vi "Initialize State.vi"(8 "error in (no error)":errorcluster, 11 "Elevator Controller in":refnum<class "Elevator Controller.lvclass">) -> (0 "error out":errorcluster, 3 "Elevator Controller out":refnum<class "Elevator Controller.lvclass">)   [LabVIEW 2019]
uses:
  Abstract Display Console Actor/Abstract Display Console Messages/Initialize Display State Msg/Initialize Display State Msg.lvclass
  Abstract Sensor Interface Actor/Abstract Sensor Interface Messages/Initalize Sensor Interface State Msg/Initalize Sensor Interface State Msg.lvclass
  Abstract User Console Actor/Abstract User Console Messages/Initialize User Console State Msg/Initialize User Console State Msg.lvclass
  <vilib>/ActorFramework/Message Enqueuer/Message Enqueuer.lvclass
  Elevator Controller.lvclass
  C:/Program Files (x86)/National Instruments/LabVIEW 2019/vi.lib/ActorFramework/Actor/Actor.lvclass
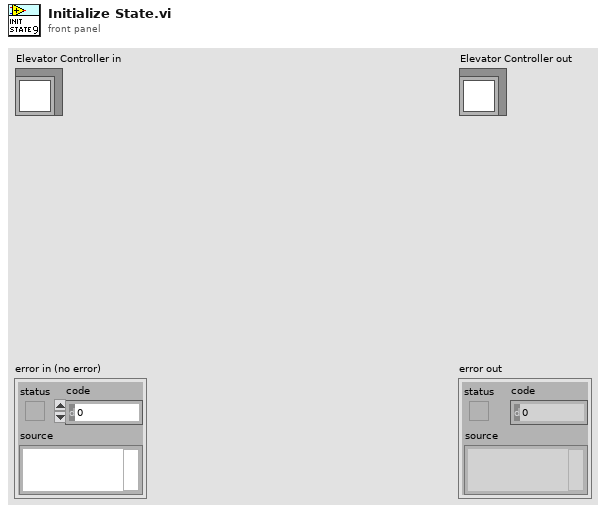
[diagram p1: front panel]
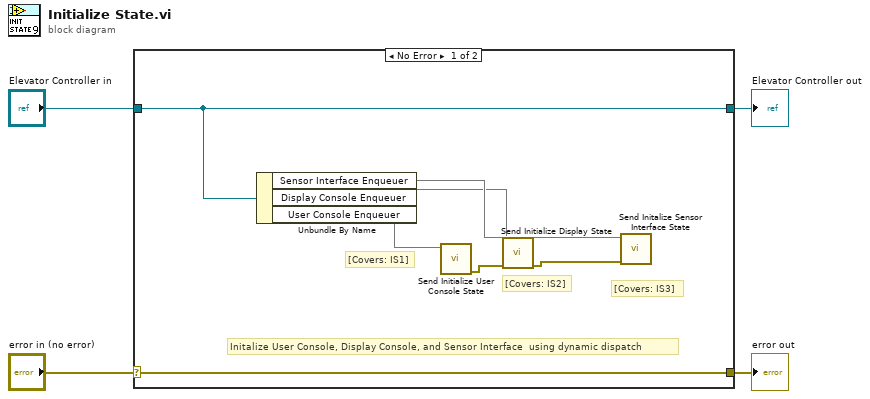
[diagram p0: block diagram]
diagram:
  n1 = case shown="No Error" "error in (no error)" {
    selector: "error in (no error)" -> [w11 w13]
    tunnel: [w11 w13] -> w3
    tunnel: [w5 w12] -> w1
    tunnel: "Elevator Controller in" -> [w5 w12]
    frame No Error {
      # "Initalize User Console, Display Console, and Sensor Interface  using dynamic dispatch"
      # "[Covers: IS2]"
      # "[Covers: IS1]"
      # "[Covers: IS3]"
      n2 = Unbundle By Name(w5) -> ("Sensor Interface Enqueuer"=w7, "Display Console Enqueuer"=w6, "User Console Enqueuer"=w10)
      n3 = call "Send Initialize User Console State.vi"("Message Enqueuer"=w10) -> ("error out"=w9:errorcluster)  [unwired: 9 in, 1 out]
      n4 = call "Send Initialize Display State.vi"("error in (no error)"=w9, "Message Enqueuer"=w6) -> ("error out"=w8:errorcluster)  [unwired: 8 in, 1 out]
      n5 = call "Send Initalize Sensor Interface State.vi"("error in (no error)"=w8, "Message Enqueuer"=w7) -> ()  [unwired: 8 in, 2 out]
    }
    frame Error {
    }
  }
  "error out" <- w3
  "Elevator Controller out" <- w1
